vi "Restart Timer.vi"(8 "error in (no error)":errorcluster, 11 "Model in":refnum<class "Model.lvclass">) -> (0 "error out":errorcluster, 3 "Model out":refnum<class "Model.lvclass">)   [LabVIEW 2016]
uses:
  Model.lvclass
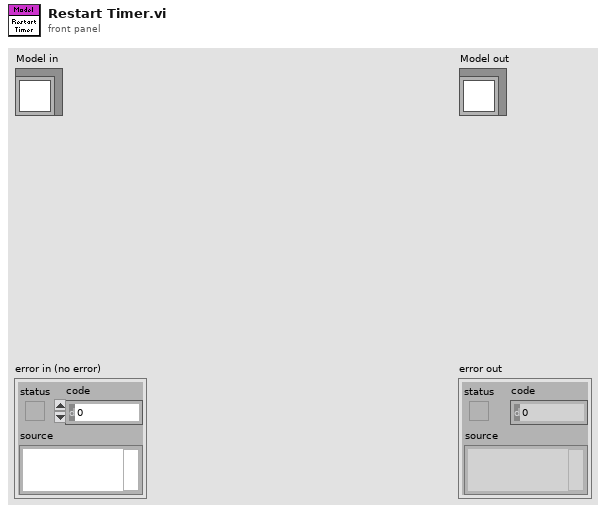
[diagram p1: front panel]
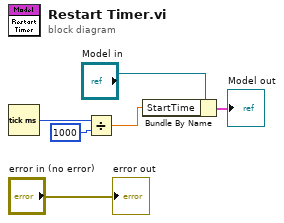
[diagram p0: block diagram]
diagram:
  n1 = Tick Count (ms)() -> (millisecond timer value=w2:u32)
  n2 = Divide(x=w2, y=u32 1000 ("x")) -> (x/y=w1:dbl)
  n3 = Bundle By Name(cluster="Model in", "StartTime"=w1) -> (→"Model out":cluster{})
  "error out" <- "error in (no error)"
